vi "StartServerVi.vi"(0 "ROS in":T1={"topic port"=0, "Node"="", "topic"="", "type"="", "node port"=0, "error "={"status"=FALSE, "code"=0, "source"=""}, "Direction"=enum."Node", "APIs"=[], "Update (ms)"=1, "write queue"=1}) -> (1 "error out":errorcluster, 2 "Reply":string, 3 "ROS out":T1={"topic port"=0, "Node"="", "topic"="", "type"="", "node port"=0, "error "={"status"=FALSE, "code"=0, "source"=""}, "Direction"=enum."Node", "APIs"=[], "Update (ms)"=1, "write queue"=1})   [LabVIEW 2012]
doc: "Start a server VI for the topic. If the exists, open it. If it's running, do nothing. If it doesn't exist, create it by copying the blank server and renaming the VI."
uses:
  _ROSControl.ctl
  _ROSDirection.ctl
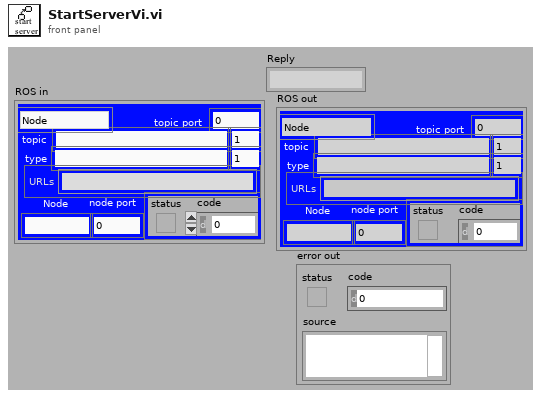
[diagram p1: front panel]
types:
  T1 = typedef "_ROSControl.ctl" = cluster{"topic port":u16, "Node":string, "topic":string, "type":string, "node port":u32, "error ":errorcluster, "Direction":T2, "APIs":string[], "Update (ms)":u16, "write queue":u16}
  T2 = typedef "_ROSDirection.ctl" = enum16{"Node", "Publisher", "Subscriber", "Service Client"}
  T3 = typedef "ServoInfo.ctl" = cluster{"vi name":string, "VI Refnum":refnum<vi>, "queue":refnum<queue>, "ROS":T1, "notifier":refnum<notifier>}
  T4 = enum32{"Bad", "Idle", "Run top level", "Running"}
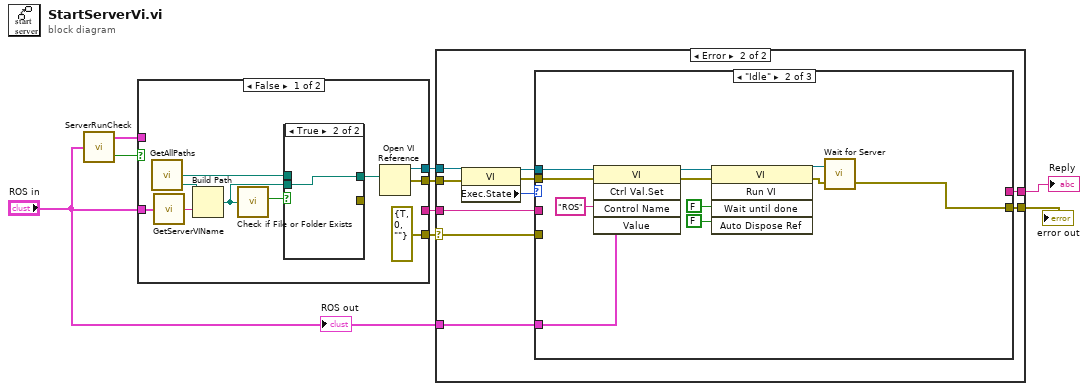
[diagram p0: block diagram]
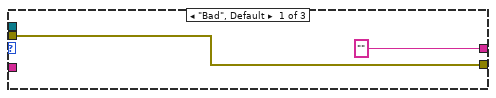
[diagram p3: hidden frame]
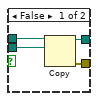
[diagram p5: hidden frame]
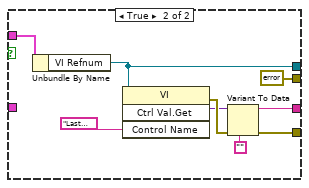
[diagram p6: hidden frame]
diagram:
  n1 = call "ServerRunCheck.vi"("ROS in"="ROS in") -> ("Running?"=w5:bool, "ServerFound"=w4:T3)
  n2 = case shown="False" w5 {
    tunnel: [w19 w28] -> w8
    tunnel: [w18 errorcluster {"status"=FALSE, "code"=0, "source"=""} ("error out")] -> w7
    tunnel: w4 -> [_ w32]
    tunnel: "ROS in" -> [w12 _]
    tunnel: [_ w26] -> w3
    tunnel: [errorcluster {"status"=TRUE, "code"=0, "source"=""} ("error out") w25] -> w2
    frame False {
      n3 = call "GetAllPaths.vi"() -> ("Server Folder"=w13:path, "BlankServer"=w14:path)  [unwired: 1 in, 1 out]
      n4 = call "GetServerVIName.vi"("ROS"=w12) -> ("vi name"=w11:string)
      n5 = Build Path(base path=w13, name or relative path=w11) -> (appended path=w16:path)
      n6 = call <vilib>:"Check if File or Folder Exists.vi"("path"=w16) -> ("file or folder exists?"=w15:bool)  [unwired: 8 in, 2 out]
      n7 = case shown="True" w15 {
        tunnel: w14 -> [w23 _]
        tunnel: w16 -> [w22 w24]
        tunnel: [w21 w24] -> w17
        tunnel: [w20 _] -> _
        frame False {
          n8 = Copy(10:w22, 11:w23) -> (0:w20:errorcluster, 3:w21:path)  [unwired: 3 in, 1 out]
        }
        frame True {
        }
      }
      n9 = Open VI Reference(vi path=w17) -> (vi reference=w19:refnum<vi>, error out=w18:errorcluster)  [unwired: 5 in]
    }
    frame True {
      n10 = Unbundle By Name(w32) -> ("VI Refnum"=w28:refnum<vi>)
      n11 = invoke class="VI" method="Ctrl Val.Get"(reference=w28, "Control Name"="Last Reply") -> (error out=w31:errorcluster, "Get Control Value Variant"=w29:variant)  [unwired: 2 in, 2 out]
      n12 = Variant To Data(error in=w31, type="" ("Control Name"), Variant=w29) -> (data=w26:string, error out=w25:errorcluster)
    }
  }
  n13 = case shown="Error" w2 {
    selector: w2 -> [w34 w36]
    tunnel: [w35 w45] -> w9
    tunnel: w8 -> [_ w44]
    tunnel: w7 -> [_ w43]
    tunnel: [w34 w39] -> w6
    tunnel: "ROS in" -> [_ w37]
    tunnel: w3 -> [w35 w38]
    frame No Error {
    }
    frame Error {
      n14 = property class="VI"(reference=w44, error in=w43) -> (reference out=w41:refnum<vi>, error out=w40:errorcluster, "Exec.State"=w42:T4)
      n15 = case shown="\"Idle\"" w42 {
        tunnel: w41 -> [_ w56 _]
        tunnel: [w47 w48 w59] -> w39
        tunnel: w40 -> [w47 w53 _]
        tunnel: w37 -> [_ w49 _]
        tunnel: ["" ("Control Name") _ w60] -> w45
        tunnel: w38 -> [_ _ w60]
        tunnel: w36 -> [_ _ w59]
        frame "Bad", Default {
        }
        frame "Idle" {
          n16 = invoke class="VI" method="Ctrl Val.Set"(reference=w56, error in=w53, "Control Name"="ROS", "Value"=w49) -> (reference out=w55:refnum<vi>, error out=w50:errorcluster)  [unwired: 1 in, 3 out]
          n17 = invoke class="VI" method="Run VI"(reference=w55, error in=w50, "Wait until done"=FALSE ("Wait Until Done"), "Auto Dispose Ref"=FALSE ("Wait Until Done")) -> (reference out=w51:refnum<vi>, error out=w52:errorcluster)  [unwired: 1 in, 3 out]
          n18 = call "Wait for Server.vi"("error in"=w52, "vi reference in"=w51) -> ("error out"=w48:errorcluster)  [unwired: 1 out]
        }
        frame "Run top level", "Running" {
        }
      }
    }
  }
  "Reply" <- w9
  "error out" <- w6
  "ROS out" <- "ROS in"
